vi "Vaportubes_oldoutputcluster.vi"() -> ()   [LabVIEW 2018]
uses:
  Global Variables.vi
panel:
  in  "index 2":i32=1
  in  "index":i32
  out "appended array":waveform(dbl)[](graph)
  in  "Temperature Task":refnum<k21>
  in  "stop":bool
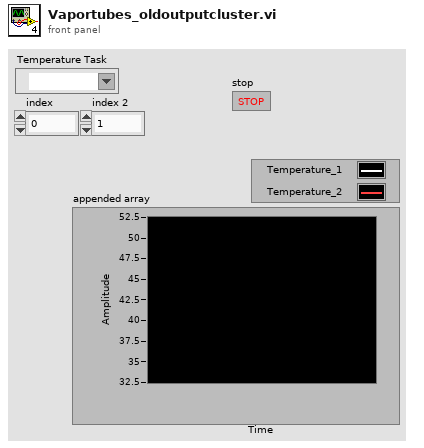
[diagram p1: front panel]
types:
  T1 = cluster{"task/channels in":refnum<k21>, "Panel Ref Out":refnum<vi>, bool}[]
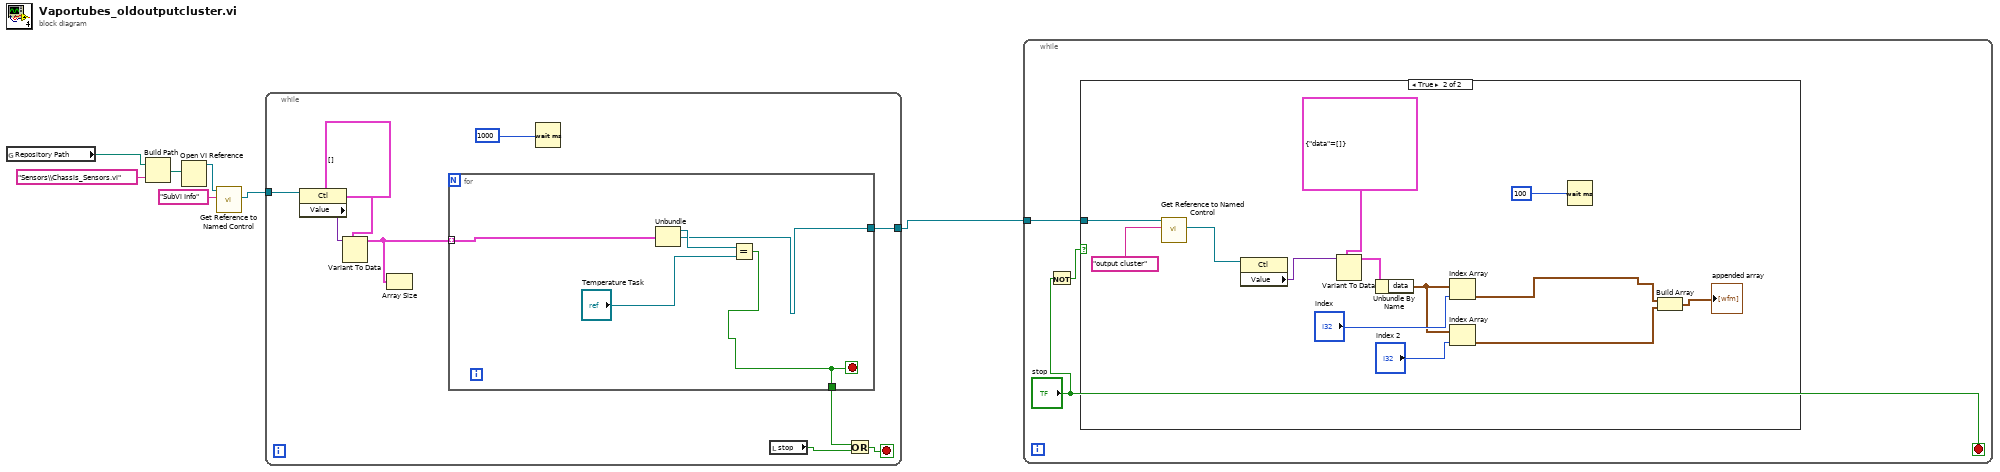
[diagram p0: block diagram]
diagram:
  n1 = global read "Global Variables.vi" "Repository Path"() -> (w2:path)
  n2 = Build Path(base path=w2, name or relative path="Sensors\\Chassis_Sensors.vi") -> (appended path=w7:path)
  n3 = Open VI Reference(vi path=w7) -> (vi reference=w5:refnum<vi>)  [unwired: 5 in, 1 out]
  n4 = call "Get Reference to Named Control.vi"("Control Name"="SubVi Info", "Front Panel Ref"=w5) -> ("Ctl Refnum"=w3:refnum<vi>)  [unwired: 7 in, 2 out]
  n5 = while {
    tunnel: w3 -> [w14]
    tunnel: [w13] -> w1
    stop <- w10 stop-if-true
    n6 = property class="Ctl"(reference=w14) -> ("Value"=w16:variant)  [unwired: 1 in, 2 out]
    n7 = Variant To Data(type=T1 [] ("SubVi Info"), Variant=w16) -> (data=w12:T1)  [unwired: 1 in, 1 out]
    n8 = Array Size(array=w12) -> ()  [unwired: 1 out]
    n9 = for {
      tunnel: w12 -> [w21] mode=indexing
      tunnel: [w18] -> w13
      tunnel: [w17] -> w9
      stop <- w17 stop-if-true
      n10 = Unbundle(w21) -> ("task/channels in"=w20:refnum<k21>, "Panel Ref Out"=w18:refnum<vi>)  [unwired: 1 out]
      n11 = Equal?(x=w20, y="Temperature Task") -> (x = y?=w17:bool)
    }
    n12 = Wait (ms)(milliseconds to wait=u32 1000) -> ()  [unwired: 1 out]
    n13 = local read "stop"() -> (w8:bool)
    n14 = Or(x=w9, y=w8) -> (x .or. y?=w10:bool)
  }
  n15 = while {
    tunnel: w1 -> [w24]
    stop <- "stop" stop-if-true
    n16 = Not(x="stop") -> (.not. x?=w22:bool)
    n17 = case shown="True" w22 {
      tunnel: w24 -> [_ w26]
      frame False {
      }
      frame True {
        n18 = call "Get Reference to Named Control.vi"("Control Name"="output cluster", "Front Panel Ref"=w26) -> ("Ctl Refnum"=w25:refnum<vi>)  [unwired: 7 in, 2 out]
        n19 = property class="Ctl"(reference=w25) -> ("Value"=w37:variant)  [unwired: 1 in, 2 out]
        n20 = Variant To Data(type=cluster{"data":waveform(dbl)[]} {"data"=[]} ("output cluster"), Variant=w37) -> (data=w34:cluster{"data":waveform(dbl)[]})  [unwired: 1 in, 1 out]
        n21 = Unbundle By Name(w34) -> ("data"=w32:waveform(dbl)[])
        n22 = Index Array(array=w32, index="index") -> (element=w29:waveform(dbl))
        n23 = Index Array(array=w32, index="index 2") -> (element=w30:waveform(dbl))
        n24 = Wait (ms)(milliseconds to wait=u32 100) -> ()  [unwired: 1 out]
        n25 = Build Array(w29, w30) -> (→"appended array":waveform(dbl)[])
      }
    }
  }
